vi "TCP Named Service - Client.vi"() -> ()   [LabVIEW 2015]
doc: "This VI implements a client for the TCP Named Service - Server.vi. It connects to a service by specifying the server address and the name of the service. The client receives the string sent by the server, displays the string and closes the connection."
panel:
  out "MirrorCoverMotor":T1
  out "Message from Server":string
  # "Overview: Demonstrates the use of the TCP functions to connect to a TCP server VI via named service and receive data.\nInstructions:\n1. Ensure TCP Named Service - Server.vi is already running.\n2. Run the VI."
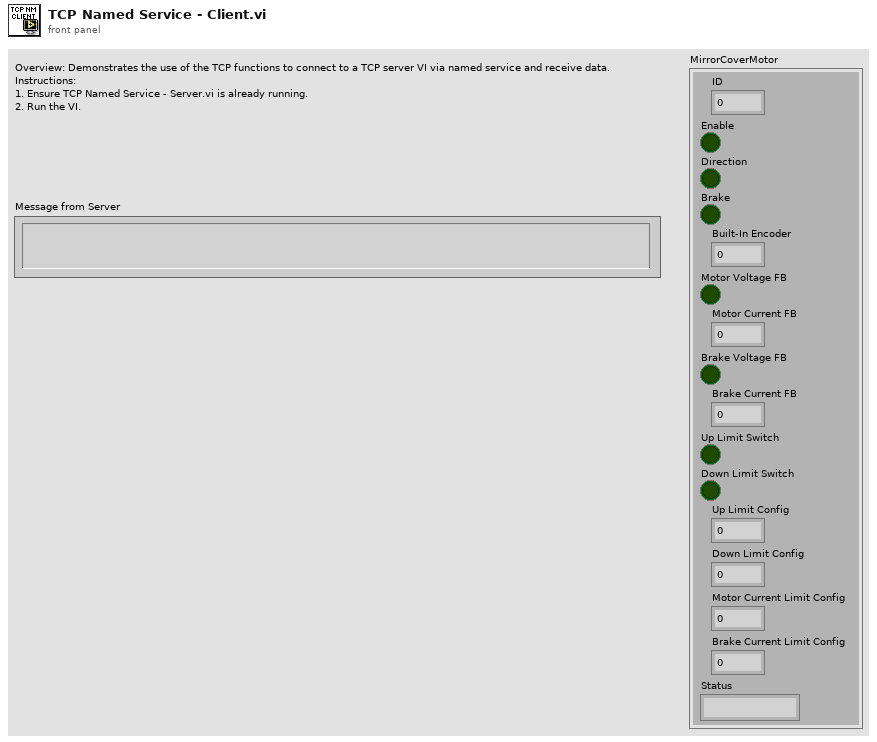
[diagram p1: front panel]
types:
  T1 = cluster{"ID":i32, "Enable":bool, "Direction":bool, "Brake":bool, "Built-In Encoder":u64, "Motor Voltage FB":bool, "Motor Current FB":u64, "Brake Voltage FB":bool, "Brake Current FB":u64, "Up Limit Switch":bool, "Down Limit Switch":bool, "Up Limit Config":u64, "Down Limit Config":u64, "Motor Current Limit Config":u64, "Brake Current Limit Config":u64, "Status":string}
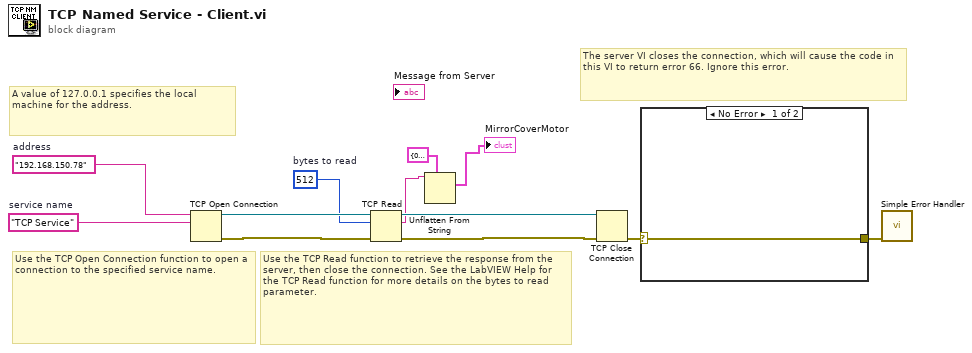
[diagram p0: block diagram]
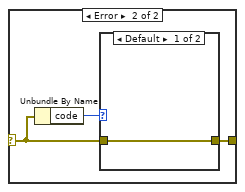
[diagram p2: hidden frame]
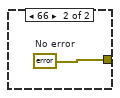
[diagram p3: hidden frame]
diagram:
  w4 = 512  # bytes to read
  w7 = "TCP Service"  # service name
  w8 = "192.168.150.78"  # address
  # "The server VI closes the connection, which will cause the code in this VI to return error 66. Ignore this error."
  # "A value of 127.0.0.1 specifies the local machine for the address."
  # "Use the TCP Open Connection function to open a connection to the specified service name."
  # "Use the TCP Read function to retrieve the response from the server, then close the connection. See the LabVIEW Help for the TCP Read function for more details on the bytes to read parameter."
  n1 = TCP Open Connection(address=w8, remote port or service name=w7) -> (connection ID=w11:refnum<k5>, error out=w12:errorcluster)  [unwired: 3 in]
  n2 = TCP Read(connection ID=w11, bytes to read=w4, error in (no error)=w12) -> (connection ID out=w10:refnum<k5>, data out=w3:string, error out=w9:errorcluster)  [unwired: 2 in]
  n3 = Unflatten From String(type=T1 {"ID"=0, "Enable"=FALSE, "Direction"=FALSE, "Brake"=FALSE, "Built-In Encoder"=0, "Motor Voltage FB"=FALSE, "Motor Current FB"=0, "Brake Voltage FB"=FALSE, "Brake Current FB"=0, "Up Limit Switch"=FALSE, "Down Limit Switch"=FALSE, "Up Limit Config"=0, "Down Limit Config"=0, "Motor Current Limit Config"=0, "Brake Current Limit Config"=0, "Status"=""} ("MirrorCoverMotor"), binary string=w3) -> (value=→"MirrorCoverMotor":T1)  [unwired: 3 in, 2 out]
  n4 = TCP Close Connection(connection ID=w10, error in (no error)=w9) -> (error out=w6:errorcluster)  [unwired: 1 in, 1 out]
  n5 = case shown="No Error" w6 {
    selector: w6 -> [w13 w15]
    tunnel: [w13 w14] -> w5
    frame No Error {
    }
    frame Error {
      n6 = Unbundle By Name(w15) -> ("code"=w16:i32)
      n7 = case shown="Default" w16 {
        tunnel: w15 -> [w17 _]
        tunnel: [w17 w18] -> w14
        frame Default {
        }
        frame 66 {
          w18 = errorcluster {"status"=FALSE, "code"=0, "source"=""}  # No error
        }
      }
    }
  }
  n8 = call <vilib>:"Simple Error Handler.vi"("error in (no error)"=w5) -> ()  [unwired: 4 in, 5 out]
